vi "VI Tree.vi"   [LabVIEW 2018, in "Keithley 3706.lvlib"]
uses:
  <instrlib>/Keithley 3706/Keithley 3706.lvlib
panel:
  # "(c) 2016 <Enter Company Name Here>.  ALL RIGHTS RESERVED."
  # "SEE DIAGRAM\nFOR VI TREE."
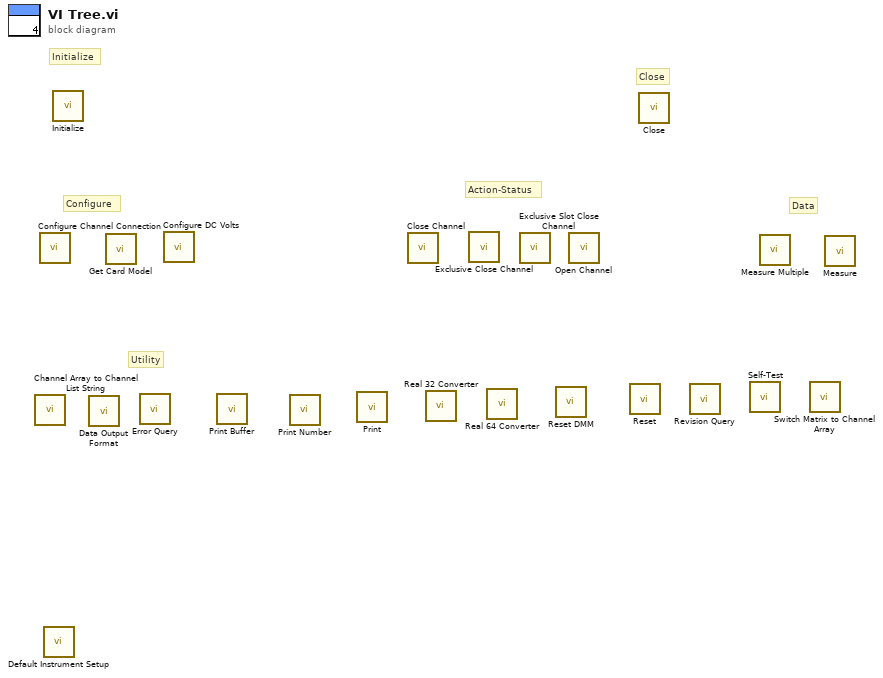
[diagram p0: block diagram]
diagram:
  # "Utility"
  # "Data"
  # "Action-Status"
  # "Configure"
  # "Close"
  # "Initialize"
  n1 = call <instrlib>:"Channel Array to Channel List String.vi"() -> ()  [unwired: 11 in, 1 out]
  n2 = call <instrlib>:"Configure Channel Connection.vi"() -> ()  [unwired: 10 in, 2 out]
  n3 = call <instrlib>:"Default Instrument Setup.vi"() -> ()  [unwired: 10 in, 2 out]
  n4 = call <instrlib>:"Initialize.vi"() -> ()  [unwired: 10 in, 2 out]
  n5 = call <instrlib>:"Data Output Format.vi"() -> ()  [unwired: 10 in, 2 out]
  n6 = call <instrlib>:"Get Card Model.vi"() -> ()  [unwired: 9 in, 3 out]
  n7 = call <instrlib>:"Error Query.vi"() -> ()  [unwired: 8 in, 4 out]
  n8 = call <instrlib>:"Configure DC Volts.vi"() -> ()  [unwired: 9 in, 3 out]
  n9 = call <instrlib>:"Print Buffer.vi"() -> ()  [unwired: 7 in, 5 out]
  n10 = call <instrlib>:"Print Number.vi"() -> ()  [unwired: 8 in, 4 out]
  n11 = call <instrlib>:"Print.vi"() -> ()  [unwired: 8 in, 4 out]
  n12 = call <instrlib>:"Close Channel.vi"() -> ()  [unwired: 10 in, 2 out]
  n13 = call <instrlib>:"Real 32 Converter.vi"() -> ()  [unwired: 10 in, 2 out]
  n14 = call <instrlib>:"Exclusive Close Channel.vi"() -> ()  [unwired: 10 in, 2 out]
  n15 = call <instrlib>:"Real 64 Converter.vi"() -> ()  [unwired: 10 in, 2 out]
  n16 = call <instrlib>:"Exclusive Slot Close Channel.vi"() -> ()  [unwired: 10 in, 2 out]
  n17 = call <instrlib>:"Reset DMM.vi"() -> ()  [unwired: 9 in, 3 out]
  n18 = call <instrlib>:"Open Channel.vi"() -> ()  [unwired: 10 in, 2 out]
  n19 = call <instrlib>:"Reset.vi"() -> ()  [unwired: 10 in, 2 out]
  n20 = call <instrlib>:"Close.vi"() -> ()  [unwired: 11 in, 1 out]
  n21 = call <instrlib>:"Revision Query.vi"() -> ()  [unwired: 8 in, 4 out]
  n22 = call <instrlib>:"Self-Test.vi"() -> ()  [unwired: 8 in, 4 out]
  n23 = call <instrlib>:"Measure Multiple.vi"() -> ()  [unwired: 9 in, 3 out]
  n24 = call <instrlib>:"Switch Matrix to Channel Array.vi"() -> ()  [unwired: 11 in, 1 out]
  n25 = call <instrlib>:"Measure.vi"() -> ()  [unwired: 9 in, 3 out]
